vi "checkJoy.vi"() -> ()   [LabVIEW 2014]
uses:
  <vilib>/Utility/inputDevices.llb/joystickAcquire.vi
  <vilib>/Utility/inputDevices.llb/closeJoystick.vi
panel:
  in  "stop":bool
  in  "milliseconds to wait":u32
  out "error out":errorcluster
  in  "device index":i32
  out "mouse info":T1(array[cluster])
  out "key info":T2(array[cluster])
  out "joystick info":T3(array[cluster])
  out "direction info":T4
  out "button info":T5
  out "axis info":T6
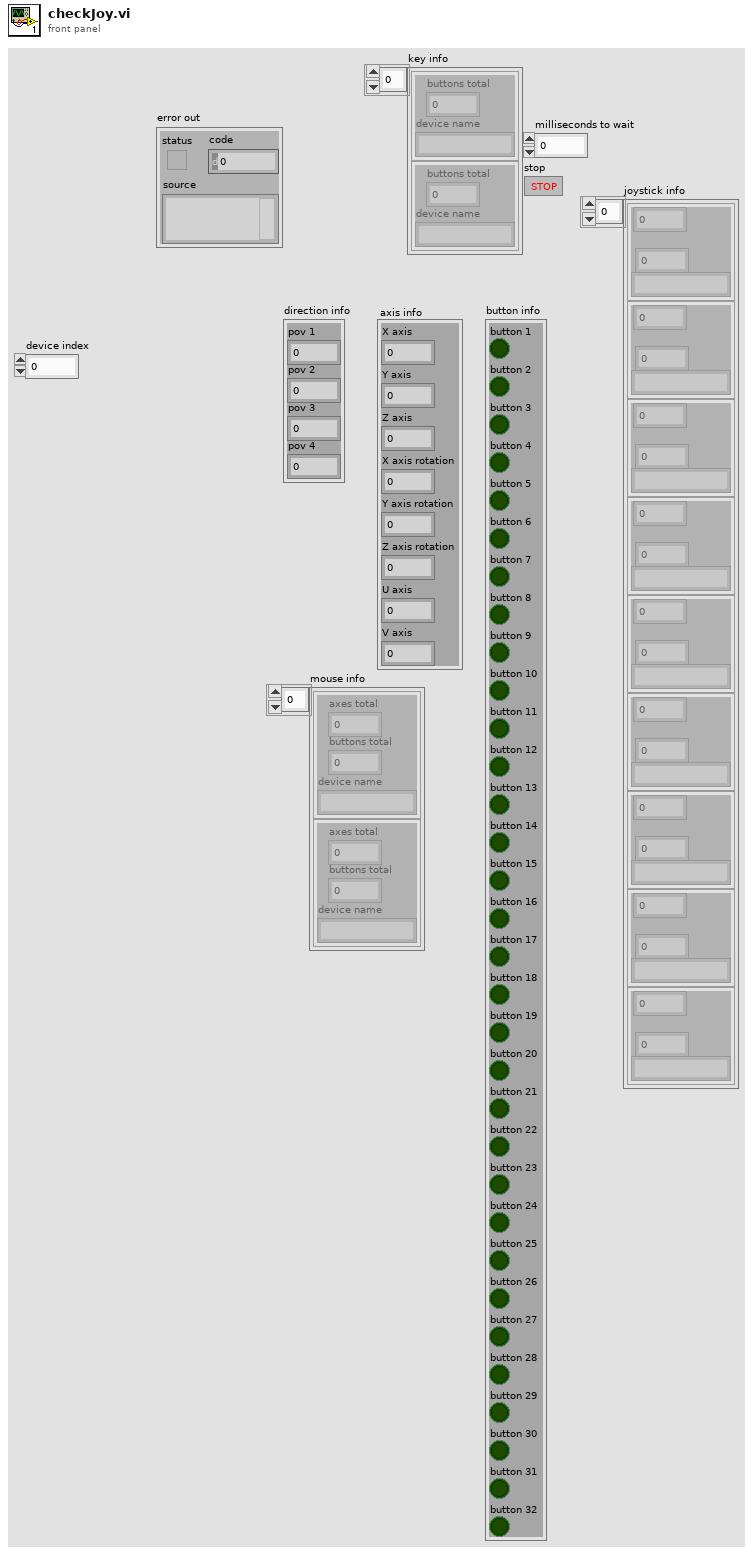
[diagram p1: front panel]
types:
  T1 = cluster{"axes total":u32, "buttons total":u32, "device name":string}[]
  T2 = cluster{"buttons total":u32, "device name":string}[]
  T3 = cluster{"axes total":u32, "buttons total":u32, "pov total":u32, "device name":string}[]
  T4 = cluster{"pov 1":i32, "pov 2":i32, "pov 3":i32, "pov 4":i32}
  T5 = cluster{"button 1":bool, "button 2":bool, "button 3":bool, "button 4":bool, "button 5":bool, "button 6":bool, "button 7":bool, "button 8":bool, "button 9":bool, "button 10":bool, "button 11":bool, "button 12":bool, "button 13":bool, "button 14":bool, "button 15":bool, "button 16":bool, "button 17":bool, "button 18":bool, "button 19":bool, "button 20":bool, "button 21":bool, "button 22":bool, "button 23":bool, "button 24":bool, "button 25":bool, "button 26":bool, "button 27":bool, "button 28":bool, "button 29":bool, "button 30":bool, "button 31":bool, "button 32":bool}
  T6 = cluster{"X axis":i32, "Y axis":i32, "Z axis":i32, "X axis rotation":i32, "Y axis rotation":i32, "Z axis rotation":i32, "U axis":i32, "V axis":i32}
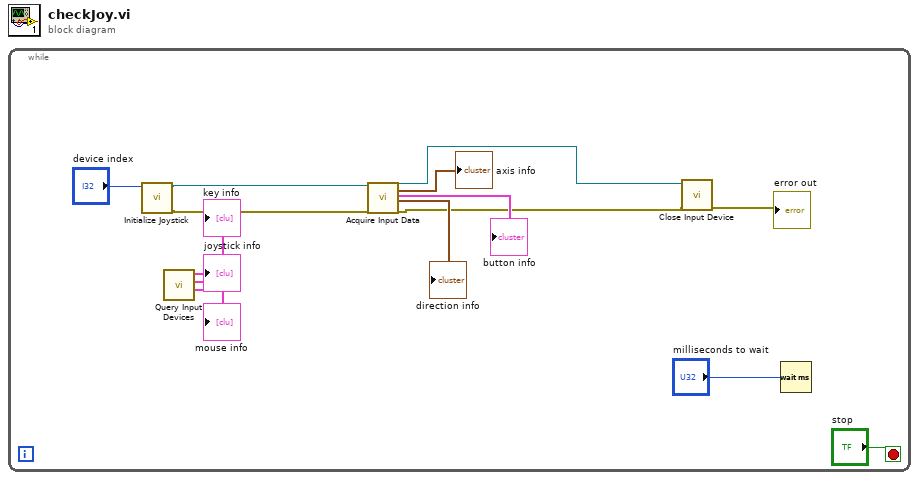
[diagram p0: block diagram]
diagram:
  n1 = while {
    stop <- "stop" stop-if-true
    n2 = call <vilib>:"Initialize Joystick.vi"("device index"="device index") -> ("error out"=w8:errorcluster, "device ID"=w7:refnum<k1>)  [unwired: 9 in]
    n3 = call <vilib>:"Query Input Devices.vi"() -> ("mouse info"=→"mouse info":T1, "key info"=→"key info":T2, "joystick info"=→"joystick info":T3)  [unwired: 8 in, 1 out]
    n4 = call-poly <vilib>:"Acquire Input Data.vi"("device ID"=w7, "error in (no error)"=w8) -> ("device ID"=w6:refnum<k1>, "axis info"=→"axis info":T6, "button info"=→"button info":T5, "direction info"=→"direction info":T4, "error out"=w5:errorcluster)  [unwired: 13 in]
    n5 = call-poly <vilib>:"Close Input Device.vi"("error in (no error)"=w5, "device ID"=w6) -> ("error out"=→"error out":errorcluster)  [unwired: 8 in]
    n6 = Wait (ms)(milliseconds to wait="milliseconds to wait") -> ()  [unwired: 1 out]
  }
